vi "aft_xmpl_Channel Simulation.vi"(11 "transmitted signal":cdb format="%0.2f") -> (3 "recieved signal":cdb)   [LabVIEW 2019]
uses:
  <vilib>/Analysis/baseanly.llb/Unit Vector (DBL).vi
  <vilib>/Analysis/NI_AALBase.lvlib
  <vilib>/ptbypt/NI_PtbyPt.lvlib
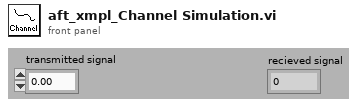
[diagram p1: front panel]
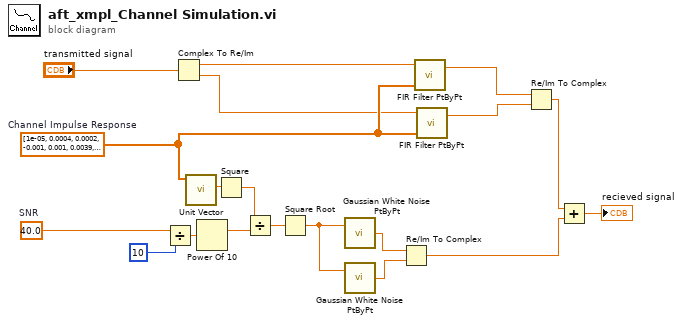
[diagram p0: block diagram]
diagram:
  w13 = 40.0  # SNR
  w6 = dbl[] [1e-05, 0.0004, 0.0002, -0.001, 0.001, 0.0039, -0.012, -0.03, -0.18, -0.1, -0.03, 0.002, 0.02, 0.05, 0.095, -0.02, -0.35, -0.3, -0.1, 0.397, 0.35, -0.03, -0.18, -0.0223, -0.01, 2.05e-05, -3.9e-07, -1.7e-08, 2e-07, 1e-06, 1e-08]  # Channel Impulse Response
  n1 = Divide(x=w13, y=10) -> (x/y=w18:dbl)
  n2 = Complex To Re/Im(x + iy="transmitted signal") -> (x=w5:dbl, y=w4:dbl)
  n3 = call-poly <vilib>:"Unit Vector.vi"("Input Vector"=w6) -> ("norm"=w19:dbl)  [unwired: 2 in, 8 out]
  n4 = Power Of 10(x=w18) -> (10^x=w15:dbl)
  n5 = Square(x=w19) -> (x^2=w16:dbl)
  n6 = Divide(x=w16, y=w15) -> (x/y=w14:dbl)
  n7 = Square Root(x=w14) -> (sqrt(x)=w3:dbl)
  n8 = call <vilib>:"Gaussian White Noise PtByPt.vi"("standard deviation"=w3) -> ("Gaussian white noise"=w12:dbl)  [unwired: 2 in]
  n9 = call <vilib>:"Gaussian White Noise PtByPt.vi"("standard deviation"=w3) -> ("Gaussian white noise"=w11:dbl)  [unwired: 2 in]
  n10 = Re/Im To Complex(1:w11, 2:w12) -> (0:w8:cdb)
  n11 = call <vilib>:"FIR Filter PtByPt.vi"("Forward Coefficients"=w6, "x"=w5) -> ("Filtered x"=w2:dbl)  [unwired: 1 in, 2 out]
  n12 = call <vilib>:"FIR Filter PtByPt.vi"("Forward Coefficients"=w6, "x"=w4) -> ("Filtered x"=w1:dbl)  [unwired: 1 in, 2 out]
  n13 = Re/Im To Complex(1:w1, 2:w2) -> (0:w9:cdb)
  n14 = Add(x=w9, y=w8) -> (x+y=→"recieved signal":cdb)
